vi "PRN Generation.vi"(8 "error in (no error)":errorcluster, 10 "Ref Data":T1={"Ass. Sensor Select"={"Ass. Sensor Select"=FALSE, "Camera-1 \nProg No."=0, "Camera-2 \nProg No."=0, "Gun \nProg No."=0}, "Torque Sensor Select"={"Torque Sensor-1"=FALSE, "Torque Sensor-2"=FALSE, "Torque Sensor-3"=FALSE, "Torque Sensor-4"=FALSE, "Torque Sensor-5"=FALSE, "Torque Sensor-6"=FALSE, "Torque Sensor-7"=FALSE, "Torque Sensor-8"=FALSE, "Torque Sensor-9"=FALSE, "Torque Sensor-10"=FALSE, "Torque Sensor-11"=FALSE, "Torque Sensor-12"=FALSE}, "Bin Seq. Select"={"First Bin"=0, "Second Bin"=0, "Third Bin"=0, "Fourth Bin"=0, "Fifth Bin"=0, "Sixth Bin"=0, "Seventh Bin"=0, "Eighth Bin"=0, "Camera-1 Trig"=0, "Camera-2 Trig"=0}, "T-Bin Seq. Select"={"First"=0, "Second"=0, "Third"=0, "Fourth"=0, "Fifth"=0, "Sixth"=0}, "Reference Barcode"={"Spring Barcode"="", "Body Barcode"="", "14 Char of Barcode"="", "Final Barcode Length"="26"}, "Label Data"={"Cust. Part No."="", "TML Part No."="", "Vendor Code"="", "Revision Level"="", "Part Description"="", "Vendor Name"=""}} {"T-Bin Seq. Select"."First" max=8 step=1; "T-Bin Seq. Select"."Second" max=8 step=1; "T-Bin Seq. Select"."Third" max=8 step=1; "T-Bin Seq. Select"."Fourth" max=8 step=1; "T-Bin Seq. Select"."Fifth" max=8 step=1; "T-Bin Seq. Select"."Sixth" max=8; "Ass. Sensor Select"."Gun \nProg No." max=8 step=1; "Ass. Sensor Select"."Camera-2 \nProg No." max=8 step=1; "Ass. Sensor Select"."Camera-1 \nProg No." max=8 step=1}, 11 "File Name":string="PSA") -> (0 "error out":errorcluster, 3 "PRN to Print":string, 4 "Barcode":string, 5 "Printing Date":string, 6 "Serial Number":string, 7 "SN":u32)   [LabVIEW 2017]
uses:
  Controls/Recipe.ctl
  <vilib>/Utility/config.llb/Read Key (U32).vi
  <vilib>/Utility/config.llb/Read Key (String).vi
  <vilib>/Utility/config.llb/NI_LVConfig.lvlib
panel:
  # "Bin No."
  # "Bin No."
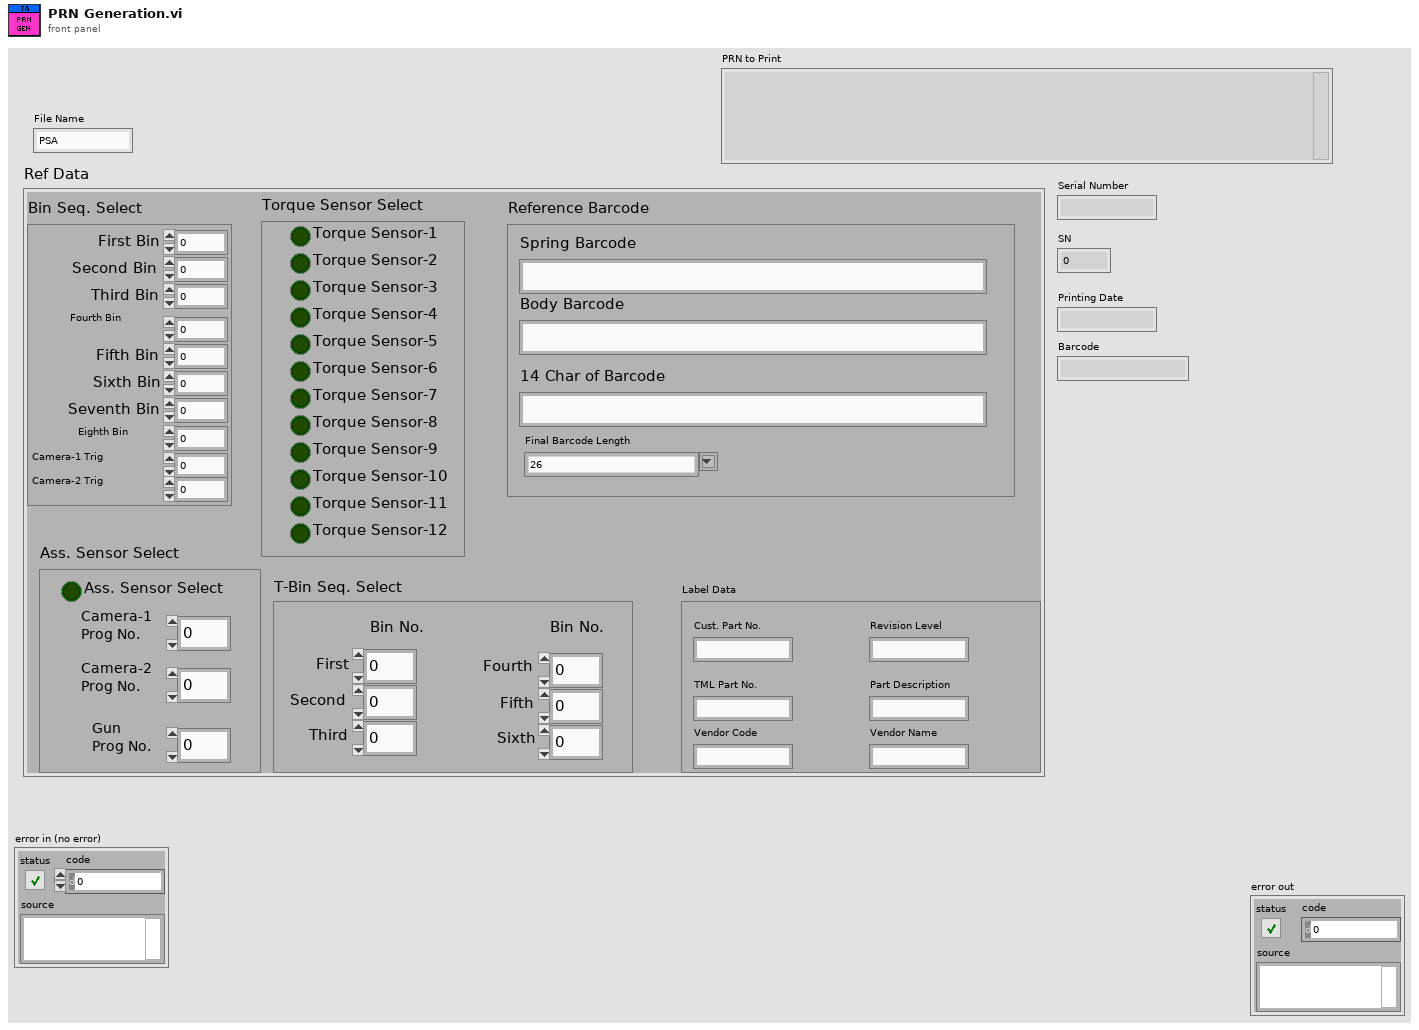
[diagram p1: front panel]
types:
  T1 = typedef "Recipe.ctl" = cluster{"Ass. Sensor Select":cluster{"Ass. Sensor Select":bool, "Camera-1 \nProg No.":u16, "Camera-2 \nProg No.":u16, "Gun \nProg No.":u16}, "Torque Sensor Select":cluster{"Torque Sensor-1":bool, "Torque Sensor-2":bool, "Torque Sensor-3":bool, "Torque Sensor-4":bool, "Torque Sensor-5":bool, "Torque Sensor-6":bool, "Torque Sensor-7":bool, "Torque Sensor-8":bool, "Torque Sensor-9":bool, "Torque Sensor-10":bool, "Torque Sensor-11":bool, "Torque Sensor-12":bool}, "Bin Seq. Select":cluster{"First Bin":u16, "Second Bin":u16, "Third Bin":u16, "Fourth Bin":u16, "Fifth Bin":u16, "Sixth Bin":u16, "Seventh Bin":u16, "Eighth Bin":u16, "Camera-1 Trig":u16, "Camera-2 Trig":u16}, "T-Bin Seq. Select":cluster{"First":u16, "Second":u16, "Third":u16, "Fourth":u16, "Fifth":u16, "Sixth":u16}, "Reference Barcode":cluster{"Spring Barcode":string, "Body Barcode":string, "14 Char of Barcode":string, "Final Barcode Length":string}, "Label Data":cluster{"Cust. Part No.":string, "TML Part No.":string, "Vendor Code":string, "Revision Level":string, "Part Description":string, "Vendor Name":string}}
  T2 = enum32{"invalid app kind", "Development System", "Run Time System", "Student Edition", "Embedded LabVIEW", "Evaluation", "Custom"}
  T3 = typedef "NI_LVConfig.lvlib/Config Data RefNum.ctl" = refnum<k1>
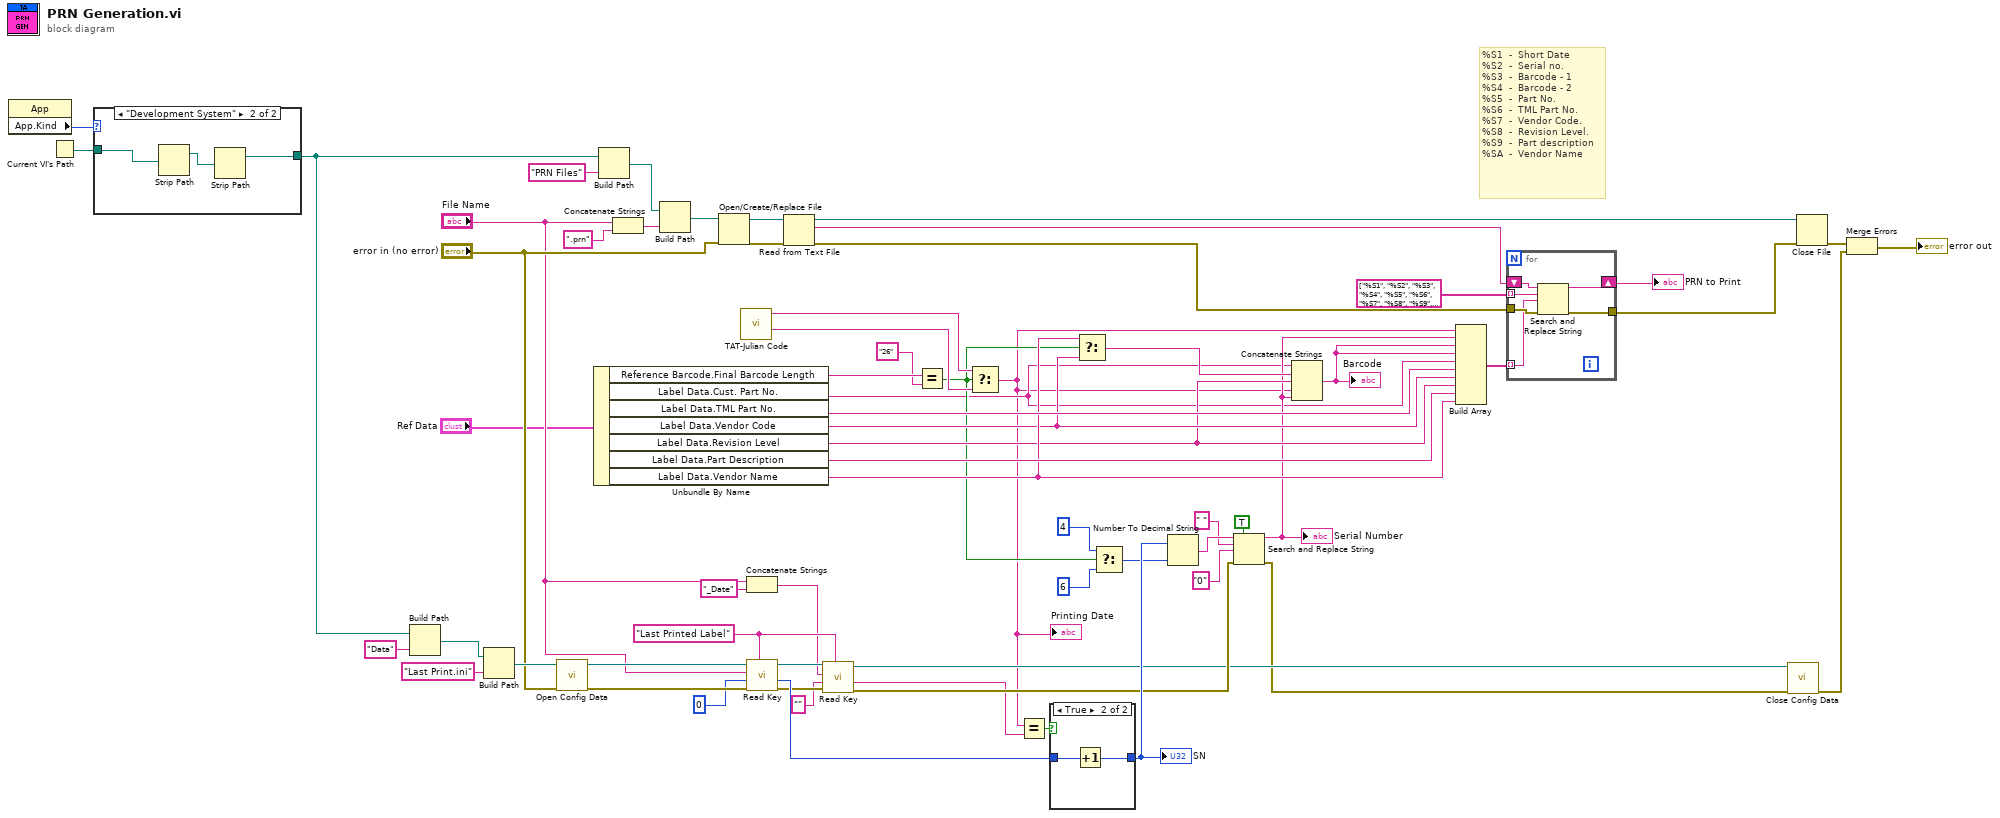
[diagram p0: block diagram]
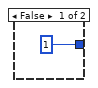
[diagram p2: hidden frame]
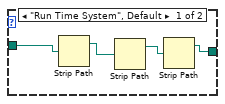
[diagram p3: hidden frame]
diagram:
  w30 = "Last Printed Label" ("section")
  # "%S1  -  Short Date\n%S2  -  Serial no.\n%S3  -  Barcode - 1\n%S4  -  Barcode - 2\n%S5  -  Part No.\n%S6  -  TML Part No.\n%S7  -  Vendor Code.\n%S8  -  Revision Level.\n%S9  -  Part description\n%SA  -  Vendor Name"
  n1 = property class="App"() -> ("App.Kind"=w57:T2)  [unwired: 2 in, 2 out]
  n2 = Current VI's Path() -> (path=w58:path)
  n3 = case shown="\"Development System\"" w57 {
    tunnel: w58 -> [w67 w71]
    tunnel: [w66 w70] -> w52
    frame "Run Time System", Default {
      n4 = Strip Path(path=w67) -> (stripped path=w69:path)  [unwired: 1 out]
      n5 = Strip Path(path=w69) -> (stripped path=w68:path)  [unwired: 1 out]
      n6 = Strip Path(path=w68) -> (stripped path=w66:path)  [unwired: 1 out]
    }
    frame "Development System" {
      n7 = Strip Path(path=w71) -> (stripped path=w72:path)  [unwired: 1 out]
      n8 = Strip Path(path=w72) -> (stripped path=w70:path)  [unwired: 1 out]
    }
  }
  n9 = Build Path(base path=w52, name or relative path="Data") -> (appended path=w53:path)
  n10 = Build Path(base path=w53, name or relative path="Last Print.ini") -> (appended path=w50:path)
  n11 = call <vilib>:"Open Config Data.vi"("error in (no error)"="error in (no error)", "configuration file path"=w50) -> ("error out"=w47:errorcluster, "refnum"=w48:T3)  [unwired: 7 in, 1 out]
  n12 = Unbundle By Name("Ref Data") -> ("Reference Barcode.Final Barcode Length"=w20:string, "Label Data.Cust. Part No."=w2:string, "Label Data.TML Part No."=w16:string, "Label Data.Vendor Code"=w11:string, "Label Data.Revision Level"=w9:string, "Label Data.Part Description"=w15:string, "Label Data.Vendor Name"=w12:string)
  n13 = Build Path(base path=w52, name or relative path="PRN Files") -> (appended path=w55:path)
  n14 = Concatenate Strings("File Name", ".prn" ("name or relative path")) -> (w64:string)
  n15 = Build Path(base path=w55, name or relative path=w64) -> (appended path=w62:path)
  n16 = Open/Create/Replace File(file path (use dialog)=w62, error in="error in (no error)") -> (refnum out=w59:refnum<file>, error out=w60:errorcluster)  [unwired: 4 in, 1 out]
  n17 = call "TAT-Julian Code.vi"() -> ("Short Date"=w17:string, "Julian Code"=w18:string)  [unwired: 8 in, 2 out]
  n18 = Concatenate Strings("File Name", "_Date" ("string")) -> (w29:string)
  n19 = call-poly <vilib>:"Read Key.vi"("section"=w30, "error in (no error)"=w47, "default value"=u32 0, "key"="File Name", "refnum"=w48) -> ("error out"=w36:errorcluster, "value"=w45:u32, "refnum out"=w37:T3)  [unwired: 3 in, 1 out]
  n20 = Read from Text File(file (use dialog)=w59, error in=w60) -> (refnum out=w61:refnum<file>, text=w28:string, error out=w26:errorcluster)  [unwired: 2 in, 1 out]
  n21 = call-poly <vilib>:"Read Key.vi"("section"=w30, "error in (no error)"=w36, "default value"="", "key"=w29, "refnum"=w37) -> ("error out"=w35:errorcluster, "value"=w3:string, "refnum out"=w14:T3)  [unwired: 3 in, 1 out]
  n22 = Equal?(x=w20, y="26") -> (x = y?=w4:bool)
  n23 = Select(t=w18, s=w4, f=w17) -> (s? t:f=w1:string)
  "Printing Date" <- w1
  n24 = Equal?(x=w1, y=w3) -> (x = y?=w31:bool)
  n25 = case shown="True" w31 {
    tunnel: w45 -> [_ w75]
    tunnel: [u32 1 w74] -> w44
    frame False {
    }
    frame True {
      n26 = Increment(x=w75) -> (x+1=w74:u32)
    }
  }
  "SN" <- w44
  n27 = Select(t=w12, s=w4, f=w11) -> (s? t:f=w10:string)
  n28 = Select(t=i16 4 ("width (-)"), s=w4, f=i16 6 ("width (-)")) -> (s? t:f=w6:i16)
  n29 = Number To Decimal String(number=w44, width (-)=w6) -> (decimal integer string=w43:string)
  n30 = Search and Replace String(replace all?=TRUE ("replace all? (F)"), input string=w43, search string=" ", replace string="0" ("replace string (\"\")"), error in=w35) -> (result string=w8:string, error out=w13:errorcluster)  [unwired: 3 in, 2 out]
  "Serial Number" <- w8
  n31 = Concatenate Strings(w2, w10, w9, w1, w8) -> (w23:string)
  "Barcode" <- w23
  n32 = Build Array(w1, w8, w23, w23, w2, w16, w11, w9, w15, w12) -> (w22:string[])
  n33 = for {
    shift-right: [w80] -> w27
    shift-left: w28 -> [w81]
    tunnel: w26 -> [w79]
    tunnel: [w78] -> w25
    tunnel: string[] ["%S1", "%S2", "%S3", "%S4", "%S5", "%S6", "%S7", "%S8", "%S9", "%SA"] -> [w77] mode=indexing
    tunnel: w22 -> [w76] mode=indexing
    n34 = Search and Replace String(input string=w81, search string=w77, replace string=w76, error in=w79) -> (result string=w80:string, error out=w78:errorcluster)  [unwired: 4 in, 2 out]
  }
  "PRN to Print" <- w27
  n35 = call <vilib>:"Close Config Data.vi"("error in (no error)"=w13, "refnum"=w14) -> ("error out"=w38:errorcluster)  [unwired: 8 in, 1 out]
  n36 = Close File(refnum=w61, error in=w25) -> (error out=w63:errorcluster)  [unwired: 1 out]
  n37 = Merge Errors(w63, w38) -> (→"error out":errorcluster)
